vi "UIProccessDriveJoysticks.vi"(9 "Axes 2":dbl[](array[numeric]), 10 "Axes":dbl[](array[numeric])) -> ()   [LabVIEW 2014, in "UILib.lvlib"]
uses:
  UILib.lvlib
  ChassisLib/ChassisLib.lvlib
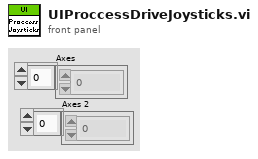
[diagram p1: front panel]
types:
  T1 = cluster{"Axes 2[0]":dbl, "Axes 2[1]":dbl, "Axes 2[2]":dbl, "Axes 2[3]":dbl, "Axes 2[4]":dbl, "Axes 2[5]":dbl, "Axes 2[6]":dbl, "Axes 2[7]":dbl, "Axes 2[8]":dbl}
  T2 = cluster{"Axes[0]":dbl, "Axes[1]":dbl, "Axes[2]":dbl, "Axes[3]":dbl, "Axes[4]":dbl, "Axes[5]":dbl, "Axes[6]":dbl, "Axes[7]":dbl, "Axes[8]":dbl}
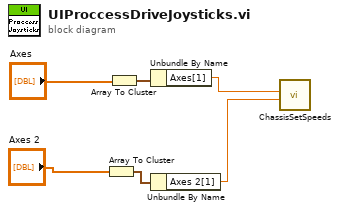
[diagram p0: block diagram]
diagram:
  n1 = Array To Cluster(array="Axes 2") -> (cluster=w3:T1)
  n2 = Array To Cluster(array="Axes") -> (cluster=w4:T2)
  n3 = Unbundle By Name(w4) -> ("Axes[1]"=w1:dbl)
  n4 = Unbundle By Name(w3) -> ("Axes 2[1]"=w2:dbl)
  n5 = call "ChassisSetSpeeds.vi"("DriveSpeedRight"=w2, "DriveSpeedLeft"=w1) -> ()  [unwired: 10 in]
